vi "fp display engine resonance.vi"(7 "channel data in":sgl[][][](array[numeric]), 10 "Image Refs In":T1[](array[typedef]), 11 "DisplayRefsIn(generic class)":refnum<vi>[](array[refnum])) -> ()   [LabVIEW 2012]
uses:
  <vilib>/vision/Image Controls.llb/IMAQ Image.ctl
  Custom Controls/Ch selector.ctl
  GFG/GFGfpRefGet.vi
  GFG/GFGbooleanGet.vi
  Custom Controls/MAIN Image panel tab Control type def.ctl
  <vilib>/vision/NI_Vision_Development_Module.lvlib
  GFG/GFG library.lvlib
panel:
  in  "ROI colors":u32[](array[colorbox])=[6618880, 16716362, 16860, 16776793, 16750848, 16448250, 16716530, 9567230, 16764108, 7340212, 32639, 0, 13816530, 8421376, 8421631, 7171459, 6618880, 16716362, 16860, 16776793, 16750848, 16448250, 16716530, 9567230, 16764108, 7340212, 32639, 0, 13816530, 8421376, 8421631, 7171459, 6618880, 16716362, 16860, 16776793, 16750848, 16448250, 16716530, 9567230, 16764108, 7340212, 32639, 0, 13816530, 8421376, 8421631, 7171459, 6618880, 16716362, 16860, 16776793, 16750848, 16448250, 16716530, 9567230, 16764108, 7340212, 32639, 0, 13816530, 8421376, 8421631, 7171459, 6618880, 16716362, 16860, 16776793, 16750848, 16448250, 16716530, 9567230, 16764108, 7340212, 32639, 0, 13816530, 8421376, 8421631, 7171459, 6618880, 16716362, 16860, 16776793, 16750848, 16448250, 16716530, 9567230, 16764108, 7340212, 32639, 0, 13816530, 8421376, 8421631, 7171459, 6618880, 16716362, 16860, 16776793, 16750848, 16448250, 16716530, 9567230, 16764108, 7340212, 32639, 0, 13816530, 8421376, 8421631, 7171459, 6618880, 16716362, 16860, 16776793, 16750848, 16448250, 16716530, 9567230, 16764108, 7340212, 32639, 0, 13816530, 8421376, 8421631, 7171459, 6618880, 16716362, 16860, 16776793, 16750848, 16448250, 16716530, 9567230, 16764108, 7340212, 32639, 0, 13816530, 8421376, 8421631, 7171459, 6618880, 16716362, 16860, 16776793, 16750848, 16448250, 16716530, 9567230, 16764108, 7340212, 32639, 0, 13816530, 8421376, 8421631, 7171459, 6618880, 16716362, 16860, 16776793, 16750848, 16448250, 16716530, 9567230, 16764108, 7340212, 32639, 0, 13816530, 8421376, 8421631, 7171459, 6618880, 16716362, 16860, 16776793, 16750848, 16448250, 16716530, 9567230, 16764108, 7340212, 32639, 0, 13816530, 8421376, 8421631, 7171459, 6618880, 16716362, 16860, 16776793, 16750848, 16448250, 16716530, 9567230, 16764108, 7340212, 32639, 0, 13816530, 8421376, 8421631, 7171459, 6618880, 16716362, 16860, 16776793, 16750848, 16448250, 16716530, 9567230, 16764108, 7340212, 32639, 0, 13816530, 8421376, 8421631, 7171459, 6618880, 16716362, 16860, 16776793, 16750848, 16448250, 16716530, 9567230, 16764108, 7340212, 32639, 0, 13816530, 8421376, 8421631, 7171459, 6618880, 16716362, 16860, 16776793, 16750848, 16448250, 16716530, 9567230, 16764108, 7340212, 32639, 0, 13816530, 8421376, 8421631, 7171459, 6618880, 16716362, 16860, 16776793, 16750848, 16448250, 16716530, 9567230, 16764108, 7340212, 32639, 0, 13816530, 8421376, 8421631, 7171459, 6618880, 16716362, 16860, 16776793, 16750848, 16448250, 16716530, 9567230, 16764108, 7340212, 32639, 0, 13816530, 8421376, 8421631, 7171459, 6618880, 16716362, 16860, 16776793, 16750848, 16448250, 16716530, 9567230, 16764108, 7340212, 32639, 0, 13816530, 8421376, 8421631, 7171459, 6618880, 16716362, 16860, 16776793, 16750848, 16448250, 16716530, 9567230, 16764108, 7340212, 32639, 0, 13816530, 8421376, 8421631, 7171459, 6618880, 16716362, 16860, 16776793, 16750848, 16448250, 16716530, 9567230, 16764108, 7340212, 32639, 0, 13816530, 8421376, 8421631, 7171459, 6618880, 16716362, 16860, 16776793, 16750848, 16448250, 16716530, 9567230, 16764108, 7340212, 32639, 0, 13816530, 8421376, 8421631, 7171459, 6618880, 16716362, 16860, 16776793, 16750848, 16448250, 16716530, 9567230, 16764108, 7340212, 32639, 0, 13816530, 8421376, 8421631, 7171459, 6618880, 16716362, 16860, 16776793, 16750848, 16448250, 16716530, 9567230, 16764108, 7340212, 32639, 0, 13816530, 8421376, 8421631, 7171459, 6618880, 16716362, 16860, 16776793, 16750848, 16448250, 16716530, 9567230, 16764108, 7340212, 32639, 0, 13816530, 8421376, 8421631, 7171459]
  out "error out":errorcluster
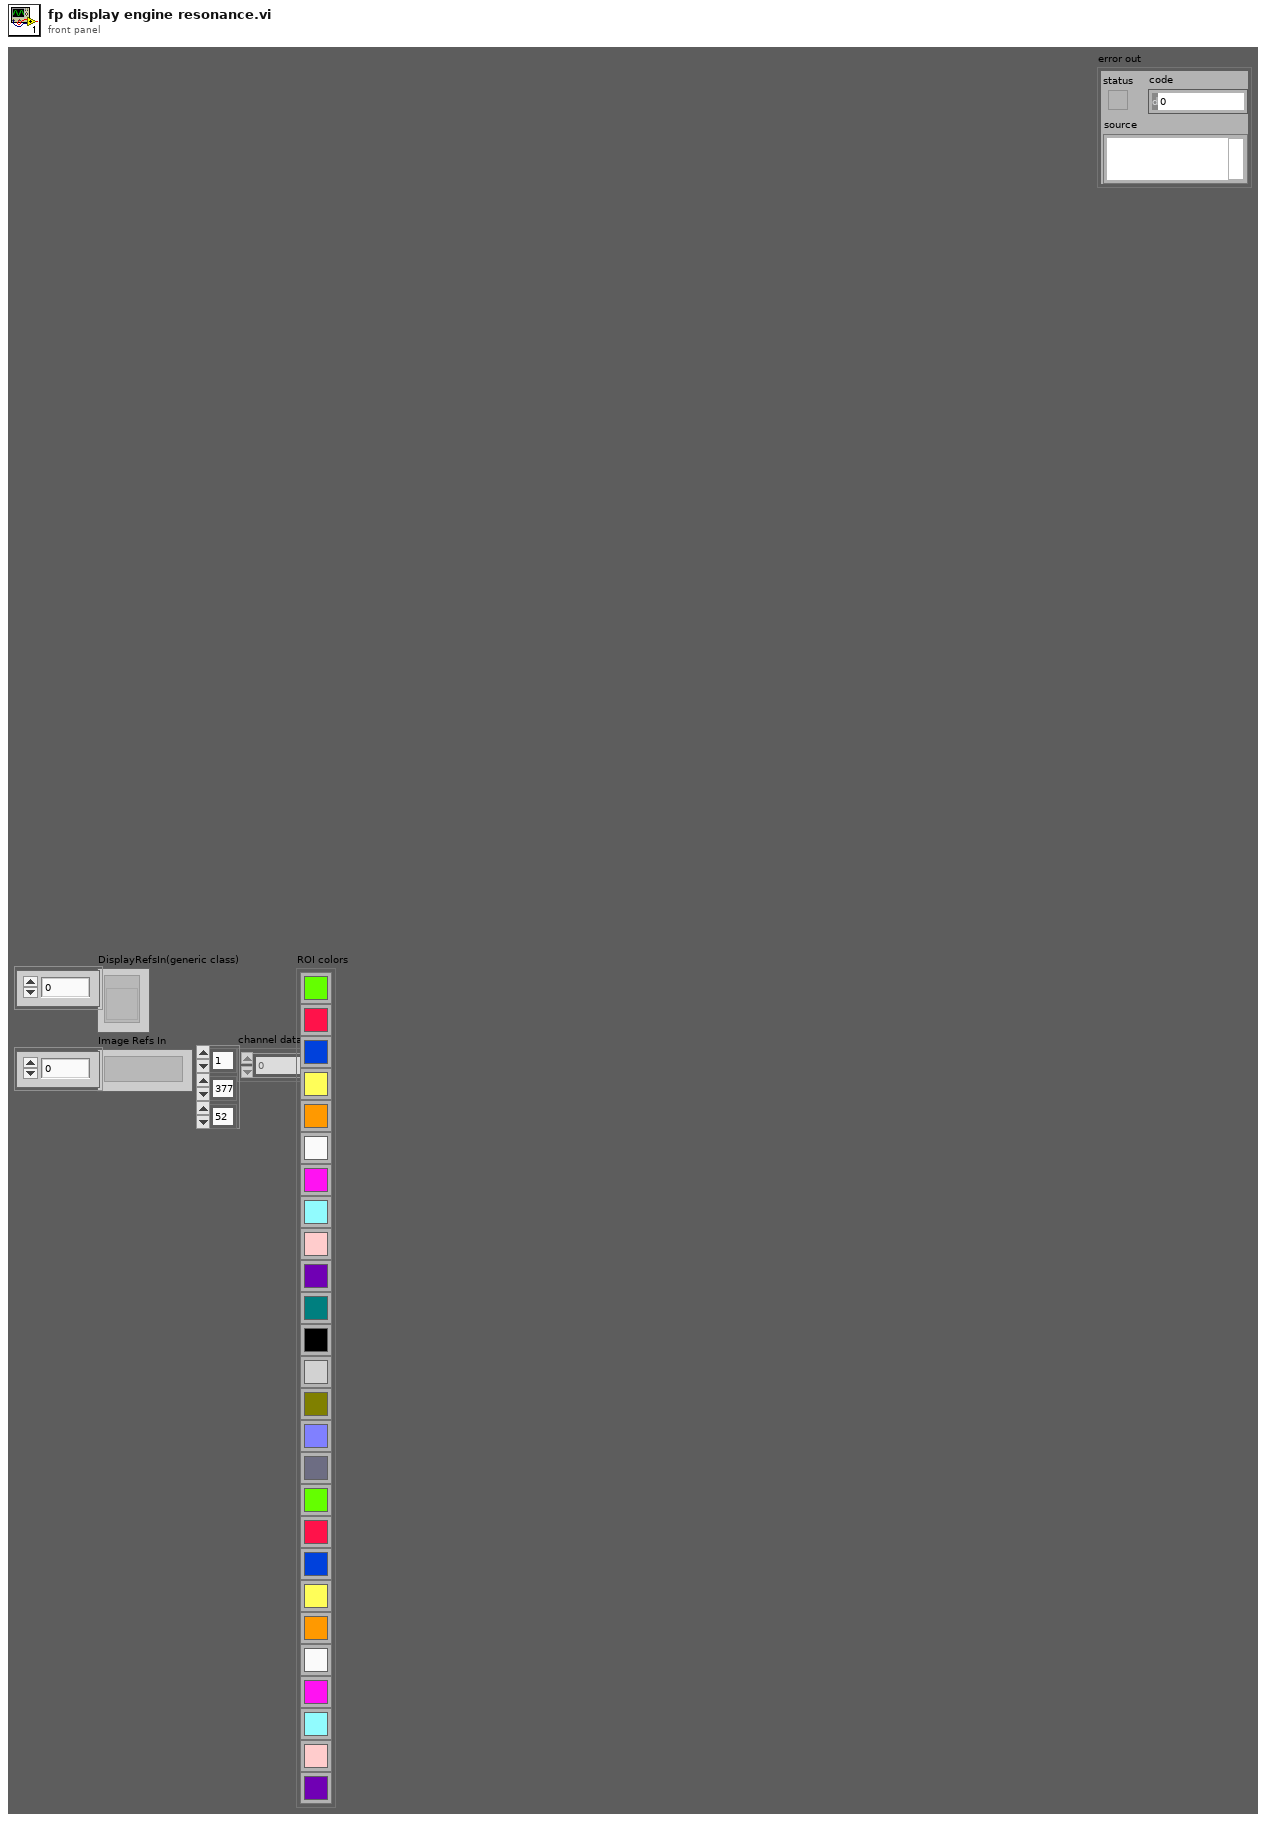
[diagram p1: front panel]
types:
  T1 = typedef "IMAQ Image.ctl" = refnum<image>
  T2 = typedef "MAIN Image panel tab Control type def.ctl" = enum32{"Channel 1", "Channel 2", "Channel 3", "Channel 4", "all channels", "RGB overlay", "ROI", "arbitrary line scan"}
  T3 = enum32{"Channel 1", "Channel 2", "Channel 3", "Channel 4", "Channel 5", "all channels", "RGB overlay", "ROI", "arbitrary line scan"}
  T4 = typedef "Ch selector.ctl" = enum16{"none", "Ch 1", "Ch 2", "Ch 3", "Ch 4", "Ch 5"}
  T5 = typedef "Image Type" = u32
  T6 = cluster{"Global Rectangle":i32[], "Contours":cluster{"Contour Type":u32, "ROI Type":u32, "Points":i32[]}[]}
  T7 = typedef "ROI Descriptor" = cluster{"Global Rectangle":i32[], "Contours":cluster{"ID":enum32{"External", "Internal"}, "Type":u32, "Coordinates":i32[]}[]}
  T8 = cluster{"WaveformChartRef":refnum<vi>, "DigitalRef":refnum<vi>, "ArrayRef":refnum<vi>, "TabControlRef":refnum<vi>, "EnumRef":refnum<vi>, "RingRef":refnum<vi>, "BooleanRef":refnum<vi>, "KnobRef":refnum<vi>, "SlideRef":refnum<vi>, "PathRef":refnum<vi>, "StringRef":refnum<vi>, "ComboBox":refnum<vi>, "WaveformGraphRef":refnum<vi>}
  T9 = cluster{"Mean Value":sgl, "Standard Variation":sgl, "Minimal Value":sgl, "Maximal Value":sgl, "Area (calibrated)":sgl, "Area (pixels)":i32, "%":sgl}[]
  T10 = cluster{"Mean Value":sgl, "Standard Variation":sgl, "Minimal Value":sgl, "Maximal Value":sgl, "Area (calibrated)":sgl, "Area (pixels)":i32, "%":sgl}
  T11 = cluster{"Contour Type":u32, "ROI Type":u32, "Points":i32[]}[]
  T12 = cluster{"Starting Value":sgl, "Incremental Value":sgl, "Histogram":u32[]}
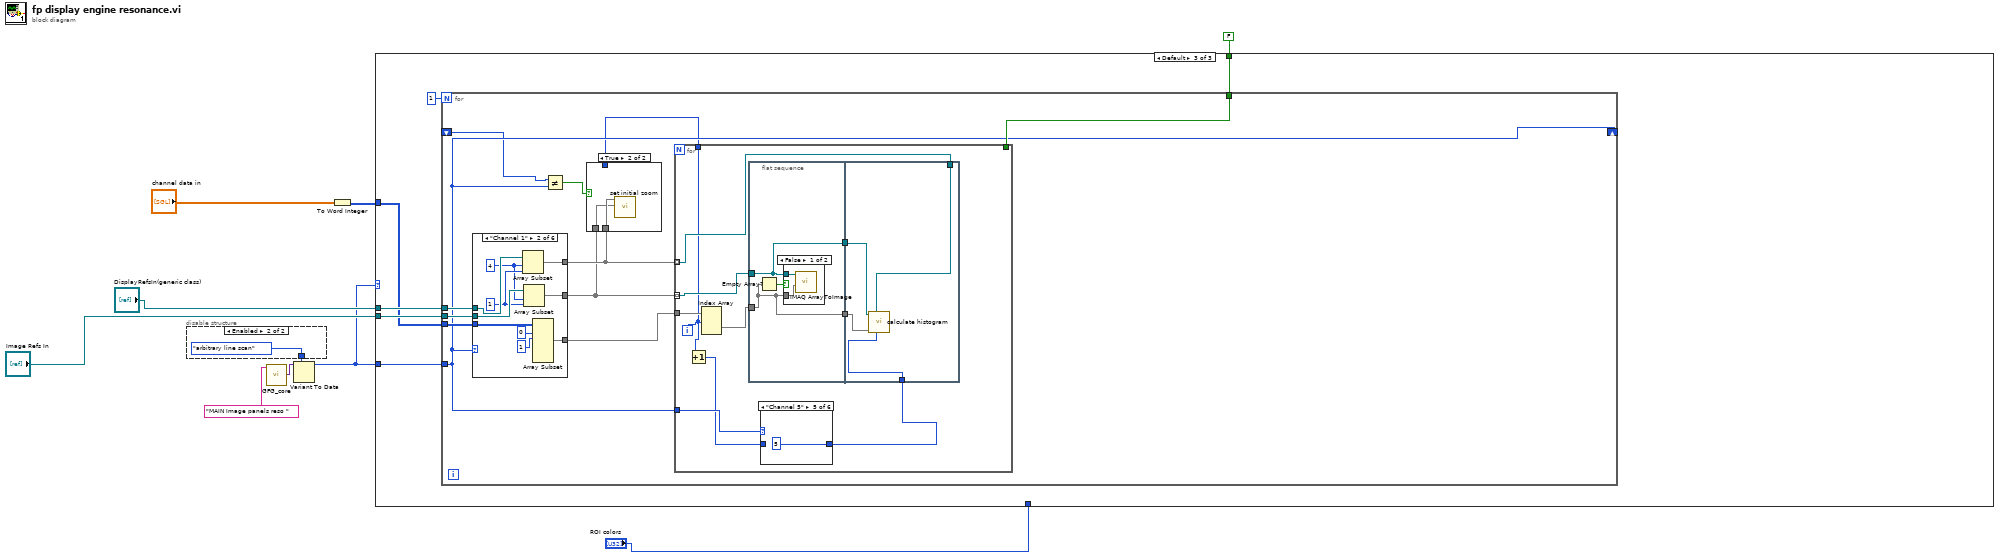
[diagram p0: block diagram]
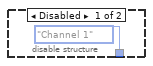
[diagram p2: hidden frame]
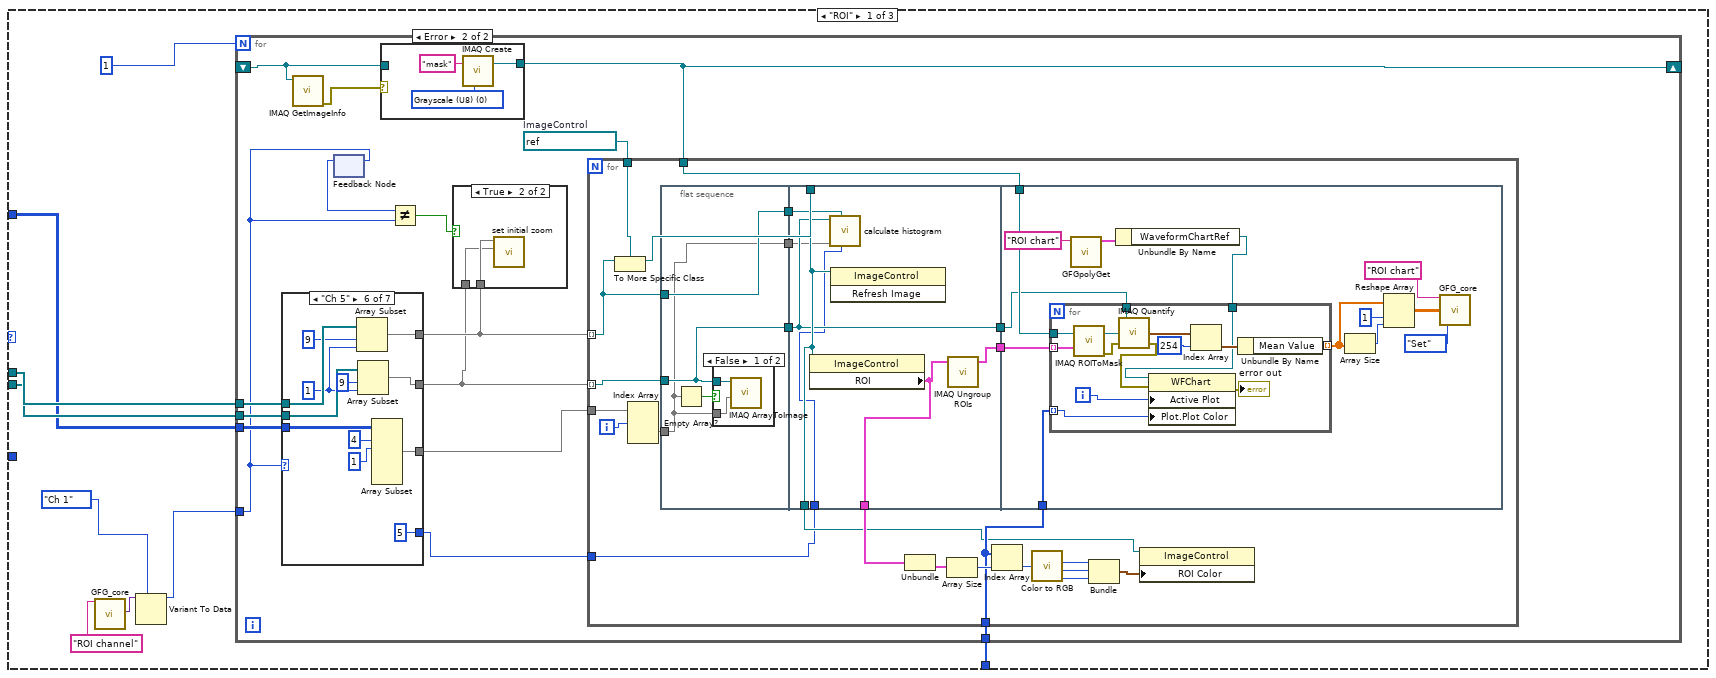
[diagram p3: hidden frame]
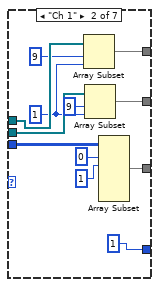
[diagram p7: hidden frame]
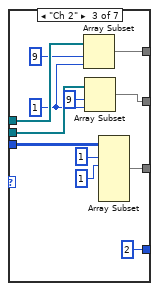
[diagram p8: hidden frame]
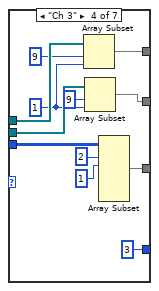
[diagram p9: hidden frame]
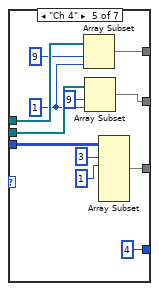
[diagram p10: hidden frame]
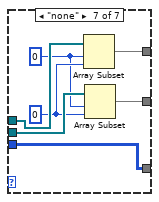
[diagram p11: hidden frame]
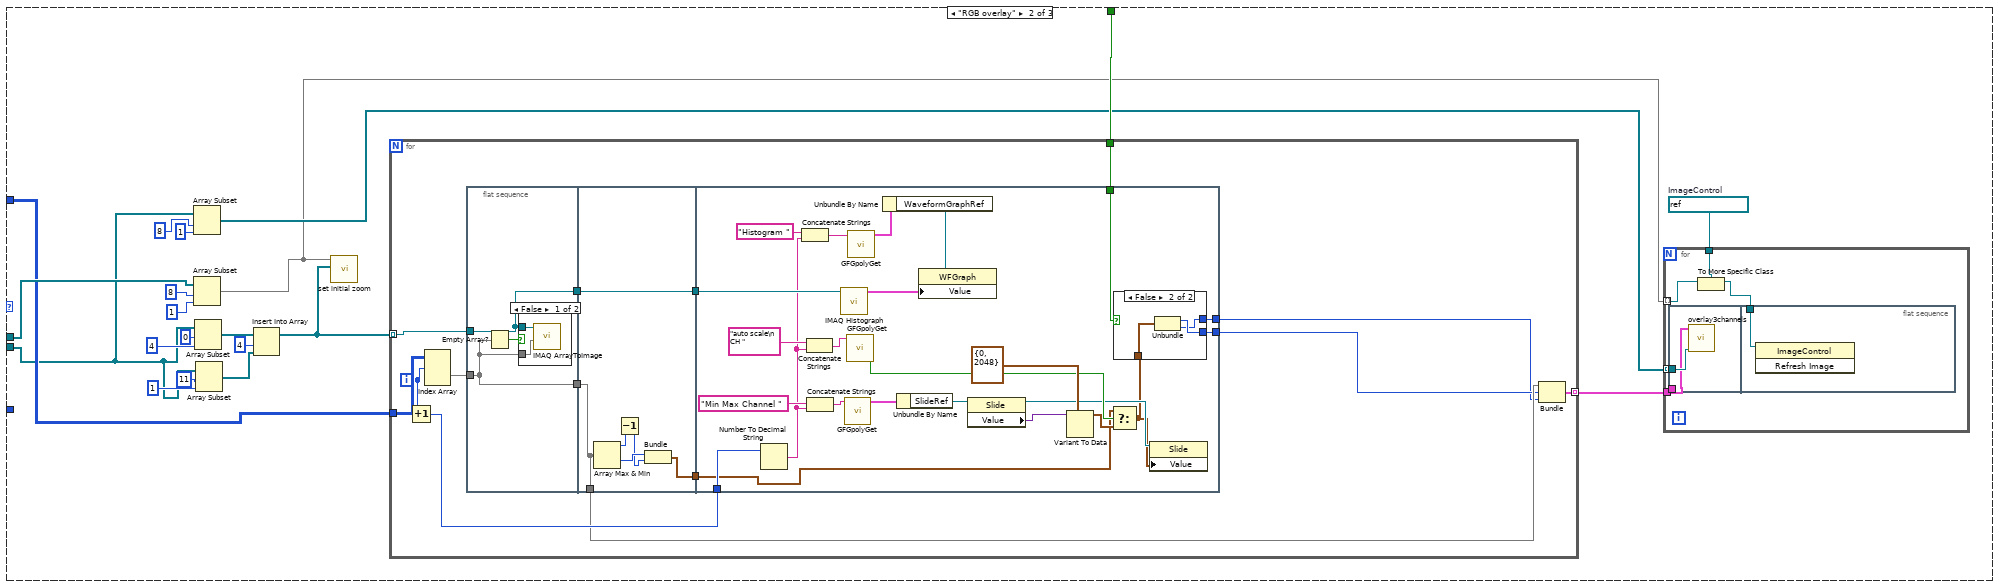
[diagram p13: hidden frame]
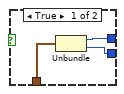
[diagram p15: hidden frame]
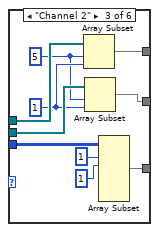
[diagram p18: hidden frame]
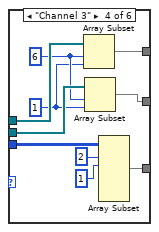
[diagram p19: hidden frame]
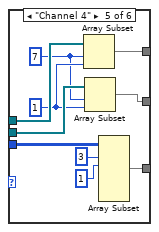
[diagram p20: hidden frame]
diagram:
  n1 = disable-structure shown="Enabled" {
    disable-tunnel: [MAIN_Image_panel_tab_Control_type_def."Channel 1" ("MAIN Image panels") T3."arbitrary line scan" ("MAIN Image panels")] -> w8
    frame Disabled {
    }
    frame Enabled {
    }
  }
  n2 = call "GFG_core.vi"("Variable Name in"="MAIN Image panels reso ") -> ("Variant Out"=w10:variant)  [unwired: 12 in, 6 out]
  n3 = Variant To Data(type=w8, Variant=w10) -> (data=w4:T3)  [unwired: 1 in, 1 out]
  n4 = To Word Integer(number="channel data in") -> (16bit integer=w3:i16[][][])
  n5 = case shown="Default" w4 {
    tunnel: w4 -> [_ _ w259]
    tunnel: "DisplayRefsIn(generic class)" -> [w20 w193 w262]
    tunnel: "Image Refs In" -> [w19 w177 w261]
    tunnel: w3 -> [w18 w192 w260]
    tunnel: FALSE -> [_ w191 w257]
    tunnel: "ROI colors" -> [w14 _ _]
    frame "ROI" {
      n6 = call "GFG_core.vi"("Variable Name in"="ROI channel") -> ("Variant Out"=w16:variant)  [unwired: 12 in, 6 out]
      n7 = Variant To Data(type=Ch_selector."Ch 1" ("ROI channel"), Variant=w16) -> (data=w15:T4)  [unwired: 1 in, 1 out]
      n8 = for {
        N: 1 -> [_]
        tunnel: w20 -> [w35]
        tunnel: w19 -> [w34]
        tunnel: w18 -> [w33]
        tunnel: w15 -> [w30]
        shift-right: [w27] -> _
        shift-left: _ -> [w26]
        tunnel: w14 -> [w24]
        w32 = refnum<vi> refnum  # ImageControl
        n9 = case shown="\"Ch 5\"" w30 {
          tunnel: w35 -> [_ w53 w65 w77 w89 w101 w108]
          tunnel: w34 -> [_ w54 w66 w78 w90 w102 w109]
          tunnel: [_ w50 w62 w74 w86 w98 w105] -> w22
          tunnel: [_ w49 w61 w73 w85 w97 w104] -> w29
          tunnel: w33 -> [_ w48 w58 w70 w82 w94 w103]
          tunnel: [_ w45 w57 w69 w81 w93 w103] -> w36
          tunnel: [_ 1 ("length") 2 ("length") 3 ("length") 4 ("length") 5 ("length") _] -> w23
          frame Default {
          }
          frame "Ch 1" {
            w52 = 1 ("length")
            n10 = Array Subset(array=w53, index=9, length=w52) -> (w49:refnum<vi>[])
            n11 = Array Subset(array=w54, index=9, length=w52) -> (w50:T1[])
            n12 = Array Subset(array=w48, index (dim 0)=0 ("index"), length (dim 0)=1 ("length")) -> (w45:i16[][][])  [unwired: 4 in]
          }
          frame "Ch 2" {
            w64 = 1 ("length")
            n13 = Array Subset(array=w65, index=9, length=w64) -> (w61:refnum<vi>[])
            n14 = Array Subset(array=w66, index=9, length=w64) -> (w62:T1[])
            n15 = Array Subset(array=w58, index (dim 0)=1 ("index"), length (dim 0)=1 ("length")) -> (w57:i16[][][])  [unwired: 4 in]
          }
          frame "Ch 3" {
            w75 = 1 ("index")
            n16 = Array Subset(array=w77, index=9, length=w75) -> (w73:refnum<vi>[])
            n17 = Array Subset(array=w78, index=9, length=w75) -> (w74:T1[])
            n18 = Array Subset(array=w70, index (dim 0)=2 ("index"), length (dim 0)=1 ("length")) -> (w69:i16[][][])  [unwired: 4 in]
          }
          frame "Ch 4" {
            w88 = 1 ("index")
            n19 = Array Subset(array=w89, index=9, length=w88) -> (w85:refnum<vi>[])
            n20 = Array Subset(array=w90, index=9, length=w88) -> (w86:T1[])
            n21 = Array Subset(array=w82, index (dim 0)=3 ("index"), length (dim 0)=1 ("length")) -> (w81:i16[][][])  [unwired: 4 in]
          }
          frame "Ch 5" {
            w100 = 1 ("index")
            n22 = Array Subset(array=w101, index=9, length=w100) -> (w97:refnum<vi>[])
            n23 = Array Subset(array=w102, index=9, length=w100) -> (w98:T1[])
            n24 = Array Subset(array=w94, index (dim 0)=4 ("index"), length (dim 0)=1 ("length")) -> (w93:i16[][][])  [unwired: 4 in]
          }
          frame "none" {
            w106 = 0 ("index")
            w107 = 0 ("length")
            n25 = Array Subset(array=w108, index=w106, length=w107) -> (w104:refnum<vi>[])
            n26 = Array Subset(array=w109, index=w106, length=w107) -> (w105:T1[])
          }
        }
        n27 = call "IMAQ GetImageInfo"("Image"=w26) -> ("error out"=w25:errorcluster)  [unwired: 3 in, 7 out]
        n28 = feedback-in #1(w30) -> ()
        n29 = feedback #1() -> (w31:T4)  [unwired: 1 in]
        n30 = case shown="Error" w25 {
          tunnel: [w37 w38] -> w27
          tunnel: w26 -> [w37 _]
          frame No Error {
          }
          frame Error {
            w39 = T5 0 items=["Grayscale (U8)", "Grayscale (I16)", "Grayscale (SGL)", "Complex (CSG)", "RGB (U32)", "HSL (U32)", "RGB (U64)"] ("Image Type")
            n31 = call "IMAQ Create"("Image Name"="mask", "Image Type"=w39) -> ("New Image"=w38:T1)  [unwired: 3 in, 1 out]
          }
        }
        n32 = Not Equal?(x=w31, y=w30) -> (x != y?=w28:bool)
        n33 = case shown="True" w28 {
          tunnel: w29 -> [_ w42]
          tunnel: w22 -> [_ w41]
          frame False {
          }
          frame True {
            n34 = call "set initial zoom.vi"("Image Refs In"=w41, "DisplayRefsIn(generic class)"=w42) -> ()  [unwired: 10 in]
          }
        }
        n35 = for {
          tunnel: w29 -> [w112] mode=indexing
          tunnel: w22 -> [w131] mode=indexing
          tunnel: w36 -> [w133]
          tunnel: w32 -> [w130]
          tunnel: w27 -> [w115]
          tunnel: w24 -> [w118]
          tunnel: w23 -> [w110]
          i -> [w128]
          n36 = To More Specific Class(target class=w130, reference=w112) -> (specific class reference=w129:refnum<vi>)  [unwired: 1 in, 1 out]
          n37 = Index Array(array=w133, index (dim 0)=w128) -> (element=w132:i16[][])  [unwired: 2 in]
          n38 = flat-sequence {
            tunnel: w132 -> [w134]
            tunnel: w131 -> [w136]
            tunnel: [w136] -> w116
            tunnel: [w135] -> w113
            tunnel: w112 -> [w135]
            tunnel: [w134] -> w111
            tunnel: w129 -> [w144]
            tunnel: [w146] -> w121
            tunnel: [w145] -> w119
            tunnel: [w142] -> w117
            tunnel: w116 -> [w142]
            tunnel: [w144] -> w114
            tunnel: w113 -> [w143]
            tunnel: w111 -> [w141]
            tunnel: w110 -> [w140]
            tunnel: w119 -> [w156]
            tunnel: w118 -> [w155]
            tunnel: w117 -> [w147]
            tunnel: w115 -> [w148]
            frame #0 {
              n39 = Empty Array?(array=w134) -> (empty?=w137:bool)
              n40 = case shown="False" w137 {
                tunnel: w136 -> [w139 _]
                tunnel: w134 -> [w138 _]
                frame False {
                  n41 = call "IMAQ ArrayToImage"("Image Pixels (I16)"=w138, "Image"=w139) -> ()  [unwired: 8 in, 2 out]
                }
                frame True {
                }
              }
            }
            frame #1 {
              n42 = property class="ImageControl"(reference=w144) -> ("ROI"=w146:T6)  [unwired: 1 in, 2 out]
              n43 = call "calculate histogram.vi"("channel no."=w140, "Image Ctrl Ref (as generic class)"=w143, "Image Array"=w141, "Image"=w142) -> ()  [unwired: 8 in]
              n44 = invoke class="ImageControl" method="Refresh Image"(reference=w144) -> ()  [unwired: 2 in, 3 out]
              n45 = call "IMAQ Ungroup ROIs"("ROI Descriptor"=w146) -> ("ROI Descriptors out"=w145:T7[])  [unwired: 3 in, 1 out]
            }
            frame #2 {
              n46 = call-poly "GFGpolyGet.vi"("Variable Name in"="ROI chart") -> ("output cluster"=w150:T8)  [unwired: 9 in, 1 out]
              n47 = Unbundle By Name(w150) -> ("WaveformChartRef"=w149:refnum<vi>)
              n48 = for {
                tunnel: w147 -> [w173]
                tunnel: w156 -> [w167] mode=indexing
                tunnel: [w169] -> w159 mode=indexing
                tunnel: w148 -> [w166]
                tunnel: w155 -> [w163] mode=indexing
                tunnel: w149 -> [w162]
                i -> [w164]
                n49 = call "IMAQ ROIToMask"("ROI Descriptor"=w167, "Image"=w166) -> ("error out"=w161:errorcluster, "Image Out"=w168:T1)  [unwired: 4 in, 1 out]
                n50 = call "IMAQ Quantify"("error in (no error)"=w161, "Image Mask"=w168, "Image"=w173) -> ("error out"=w160:errorcluster, "Region Reports"=w172:T9)  [unwired: 1 out]
                n51 = property on="Property Node" class="WFChart"(reference=w162, error in=w160, "Active Plot"=w164, "Plot.Plot Color"=w163) -> (error out=→"error out":errorcluster)  [unwired: 1 out]
                n52 = Index Array(array=w172, index=254) -> (element=w170:T10)
                n53 = Unbundle By Name(w170) -> ("Mean Value"=w169:sgl)
              }
              n54 = Array Size(array=w159) -> (size(s)=w158:i32)
              n55 = Reshape Array(w159, 1 ("dimension size"), w158) -> (w153:sgl[][])
              n56 = call "GFG_core.vi"("Variable Name in"="ROI chart", "Variant in"=w153, "Action"=enum16{"Init", "Set", "Get"}."Set") -> ()  [unwired: 10 in, 7 out]
            }
          }
          n57 = Unbundle(w121) -> ("Contours"=w126:T11)  [unwired: 1 out]
          n58 = Array Size(array=w126) -> (size(s)=w127:i32)
          n59 = Index Array(array=w118, index=w127) -> (element=w122:u32)
          n60 = call <vilib>:"Color to RGB.vi"("Color"=w122) -> ("R"=w123:u8, "G"=w124:u8, "B"=w125:u8)  [unwired: 1 out]
          n61 = Bundle("R"=w123, "G"=w124, "B"=w125) -> (w120:cluster{"R":u8, "G":u8, "B":u8})  [unwired: 1 in]
          n62 = property class="ImageControl"(reference=w114, "ROI Color"=w120) -> ()  [unwired: 1 in, 2 out]
        }
      }
    }
    frame "RGB overlay" {
      w180 = refnum<vi> refnum  # ImageControl
      n63 = Array Subset(array=w177, index=8, length=1) -> (w184:T1[])
      n64 = Array Subset(array=w193, index=8, length=1) -> (w181:refnum<vi>[])
      n65 = Array Subset(array=w177, index=0, length=4) -> (w182:T1[])
      n66 = Array Subset(array=w177, index=11, length=1) -> (w174:T1[])
      n67 = Insert Into Array(array=w182, index=4, new element=w174) -> (w176:T1[])
      n68 = call "set initial zoom.vi"("Image Refs In"=w176, "DisplayRefsIn(generic class)"=w181) -> ()  [unwired: 10 in]
      n69 = for {
        tunnel: w176 -> [w213] mode=indexing
        tunnel: w192 -> [w215]
        tunnel: w191 -> [w206]
        tunnel: [w202] -> w183 mode=indexing
        i -> [w210]
        n70 = Increment(x=w210) -> (x+1=w208:i32)
        n71 = Index Array(array=w215, index (dim 0)=w210) -> (element=w214:i16[][])  [unwired: 2 in]
        n72 = flat-sequence {
          tunnel: w214 -> [w216]
          tunnel: w213 -> [w217]
          tunnel: [w217] -> w211
          tunnel: [w216] -> w209
          tunnel: [w226] -> w212
          tunnel: w211 -> [w226]
          tunnel: w209 -> [w221]
          tunnel: [w224] -> w207
          tunnel: [w221] -> w205
          tunnel: w212 -> [w245]
          tunnel: w208 -> [w244]
          tunnel: w207 -> [w232]
          tunnel: w206 -> [w227]
          tunnel: [w229] -> w203
          tunnel: [w228] -> w204
          frame #0 {
            n73 = Empty Array?(array=w216) -> (empty?=w218:bool)
            n74 = case shown="False" w218 {
              tunnel: w217 -> [w220 _]
              tunnel: w216 -> [w219 _]
              frame False {
                n75 = call "IMAQ ArrayToImage"("Image Pixels (I16)"=w219, "Image"=w220) -> ()  [unwired: 8 in, 2 out]
              }
              frame True {
              }
            }
          }
          frame #1 {
            n76 = Array Max & Min(array=w221) -> (max value=w225:i16, min value=w223:i16)  [unwired: 2 out]
            n77 = Decrement(x=w225) -> (x-1=w222:i16)
            n78 = Bundle(w223, w222) -> (w224:cluster{i16, i16})  [unwired: 1 in]
          }
          frame #2 {
            n79 = Number To Decimal String(number=w244) -> (decimal integer string=w239:string)  [unwired: 1 in]
            n80 = Concatenate Strings("Histogram " ("string"), w239) -> (w247:string)
            n81 = Concatenate Strings("auto scale\n      CH " ("Variable Name in"), w239) -> (w242:string)
            n82 = Concatenate Strings("Min Max Channel " ("Variable Name in"), w239) -> (w230:string)
            n83 = call "IMAQ Histograph"("Image"=w245) -> ("Histogram Graph"=w250:T12)  [unwired: 7 in, 3 out]
            n84 = call-poly "GFGpolyGet.vi"("Variable Name in"=w230) -> ("output cluster"=w241:T8)  [unwired: 9 in, 1 out]
            n85 = call-poly "GFGpolyGet.vi"("Variable Name in"=w242) -> ("Boolean"=w235:bool)  [unwired: 10 in]
            n86 = call-poly "GFGpolyGet.vi"("Variable Name in"=w247) -> ("output cluster"=w248:T8)  [unwired: 9 in, 1 out]
            n87 = Unbundle By Name(w248) -> ("WaveformGraphRef"=w249:refnum<vi>)
            n88 = Unbundle By Name(w241) -> ("SlideRef"=w238:refnum<vi>)
            n89 = property class="WFGraph"(reference=w249, "Value"=w250) -> ()  [unwired: 1 in, 2 out]
            n90 = property class="Slide"(reference=w238) -> (reference out=w233:refnum<vi>, "Value"=w237:variant)  [unwired: 1 in, 1 out]
            n91 = Variant To Data(type=cluster{i32, i32} {0, 2048} ("channel1"), Variant=w237) -> (data=w234:cluster{i32, i32})  [unwired: 1 in, 1 out]
            n92 = Select(t=w232, s=w235, f=w234) -> (s? t:f=w231:cluster{i32, i32})
            n93 = case shown="False" w227 {
              tunnel: w231 -> [w253 w256]
              tunnel: [w252 w254] -> w229
              tunnel: [w251 w255] -> w228
              frame True {
                n94 = Unbundle(w253) -> (w252:i32, w251:i32)
              }
              frame False {
                n95 = Unbundle(w256) -> (w255:i32, w254:i32)
              }
            }
            n96 = property class="Slide"(reference=w233, "Value"=w231) -> ()  [unwired: 1 in, 2 out]
          }
        }
        n97 = Bundle(w205, w204, w203) -> (w202:cluster{i16[][], i32, i32})  [unwired: 1 in]
      }
      n98 = for {
        tunnel: w184 -> [w198] mode=indexing
        tunnel: w183 -> [w197]
        tunnel: w181 -> [w196] mode=indexing
        tunnel: w180 -> [w195]
        n99 = flat-sequence {
          tunnel: w198 -> [w200]
          tunnel: w197 -> [w199]
          tunnel: w194 -> [w201]
          frame #0 {
            n100 = call "overlay3channels.vi"("RGB Overlay"=w200, "Array"=w199) -> ()  [unwired: 10 in]
          }
          frame #1 {
            n101 = invoke class="ImageControl" method="Refresh Image"(reference=w201) -> ()  [unwired: 2 in, 3 out]
          }
        }
        n102 = To More Specific Class(target class=w195, reference=w196) -> (specific class reference=w194:refnum<vi>)  [unwired: 1 in, 1 out]
      }
    }
    frame Default {
      n103 = for {
        N: 1 -> [_]
        tunnel: w262 -> [w272]
        tunnel: w261 -> [w271]
        tunnel: w260 -> [w270]
        tunnel: w259 -> [w265]
        tunnel: w257 -> [w267]
        shift-right: [w265] -> _
        shift-left: _ -> [w264]
        n104 = case shown="\"Channel 1\"" w265 {
          tunnel: w272 -> [_ w284 w294 w304 w314 w324]
          tunnel: w271 -> [_ w285 w295 w305 w315 w325]
          tunnel: [_ w281 w291 w301 w311 w321] -> w266
          tunnel: [_ w280 w290 w300 w310 w320] -> w269
          tunnel: w270 -> [_ w279 w287 w297 w307 w317]
          tunnel: [_ w276 w286 w296 w306 w316] -> w273
          frame Default {
          }
          frame "Channel 1" {
            w282 = 4 ("index")
            w283 = 1 ("length")
            n105 = Array Subset(array=w284, index=w282, length=w283) -> (w280:refnum<vi>[])
            n106 = Array Subset(array=w285, index=w282, length=w283) -> (w281:T1[])
            n107 = Array Subset(array=w279, index (dim 0)=0 ("index"), length (dim 0)=1 ("length")) -> (w276:i16[][][])  [unwired: 4 in]
          }
          frame "Channel 2" {
            w292 = 5 ("index")
            w293 = 1 ("length")
            n108 = Array Subset(array=w294, index=w292, length=w293) -> (w290:refnum<vi>[])
            n109 = Array Subset(array=w295, index=w292, length=w293) -> (w291:T1[])
            n110 = Array Subset(array=w287, index (dim 0)=1 ("index"), length (dim 0)=1 ("length")) -> (w286:i16[][][])  [unwired: 4 in]
          }
          frame "Channel 3" {
            w302 = 1 ("index")
            w303 = 6 ("index")
            n111 = Array Subset(array=w304, index=w303, length=w302) -> (w300:refnum<vi>[])
            n112 = Array Subset(array=w305, index=w303, length=w302) -> (w301:T1[])
            n113 = Array Subset(array=w297, index (dim 0)=2 ("index"), length (dim 0)=1 ("length")) -> (w296:i16[][][])  [unwired: 4 in]
          }
          frame "Channel 4" {
            w312 = 7 ("index")
            w313 = 1 ("index")
            n114 = Array Subset(array=w314, index=w312, length=w313) -> (w310:refnum<vi>[])
            n115 = Array Subset(array=w315, index=w312, length=w313) -> (w311:T1[])
            n116 = Array Subset(array=w307, index (dim 0)=3 ("index"), length (dim 0)=1 ("length")) -> (w306:i16[][][])  [unwired: 4 in]
          }
          frame "Channel 5" {
            w322 = 11 ("index")
            w323 = 1 ("index")
            n117 = Array Subset(array=w324, index=w322, length=w323) -> (w320:refnum<vi>[])
            n118 = Array Subset(array=w325, index=w322, length=w323) -> (w321:T1[])
            n119 = Array Subset(array=w317, index (dim 0)=4 ("index"), length (dim 0)=1 ("length")) -> (w316:i16[][][])  [unwired: 4 in]
          }
        }
        n120 = Not Equal?(x=w264, y=w265) -> (x != y?=w268:bool)
        n121 = for {
          tunnel: w269 -> [w328] mode=indexing
          tunnel: w266 -> [w330] mode=indexing
          tunnel: w273 -> [w335]
          tunnel: w265 -> [w334]
          tunnel: w267 -> [_]
          tunnel: [w327] -> w263
          i -> [w327]
          n122 = Increment(x=w327) -> (x+1=w333:i32)
          n123 = Index Array(array=w335, index (dim 0)=w327) -> (element=w326:i16[][])  [unwired: 2 in]
          n124 = flat-sequence {
            tunnel: w326 -> [w336]
            tunnel: w330 -> [w337]
            tunnel: [w337] -> w332
            tunnel: [w336] -> w331
            tunnel: w332 -> [w342]
            tunnel: w331 -> [w344]
            tunnel: w329 -> [w343]
            tunnel: w328 -> [w341]
            frame #0 {
              n125 = Empty Array?(array=w336) -> (empty?=w338:bool)
              n126 = case shown="False" w338 {
                tunnel: w337 -> [w340 _]
                tunnel: w336 -> [w339 _]
                frame False {
                  n127 = call "IMAQ ArrayToImage"("Image Pixels (I16)"=w339, "Image"=w340) -> ()  [unwired: 8 in, 2 out]
                }
                frame True {
                }
              }
            }
            frame #1 {
              n128 = call "calculate histogram.vi"("channel no."=w343, "Image Ctrl Ref (as generic class)"=w341, "Image Array"=w344, "Image"=w342) -> ()  [unwired: 8 in]
            }
          }
          n129 = case shown="\"Channel 5\"" w334 {
            tunnel: [1 2 3 4 5 w350] -> w329
            tunnel: w333 -> [_ _ _ _ _ w350]
            frame "Channel 1", Default {
            }
            frame "Channel 2" {
            }
            frame "Channel 3" {
            }
            frame "Channel 4" {
            }
            frame "Channel 5" {
            }
            frame "all channels" {
            }
          }
        }
        n130 = case shown="True" w268 {
          tunnel: w269 -> [_ w275]
          tunnel: w266 -> [_ w274]
          tunnel: w263 -> [_ _]
          frame False {
          }
          frame True {
            n131 = call "set initial zoom.vi"("Image Refs In"=w274, "DisplayRefsIn(generic class)"=w275) -> ()  [unwired: 10 in]
          }
        }
      }
    }
  }
